vi "PWM.vi"(9 "Period (ms)":dbl=3.0, 10 "Duty Cycle":dbl format="%#_13g", 11 "Starting Tick Count":u32) -> (2 "Pwm value":bool, 3 "Starting Tick Count":u32)   [LabVIEW 2013]
doc: "Use this template to build a standard state machine design pattern. Each state executes code and determines which state to transition to. Contrast this design pattern with the User Interface Event Handler pattern, in which code executes in response to user actions. Contrast this design pattern also with the Queued Message Handler pattern, in which each message handling code can queue zero or more new messages."
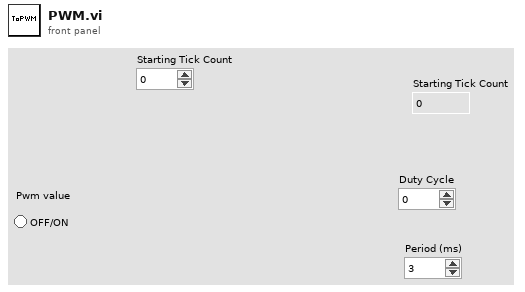
[diagram p1: front panel]
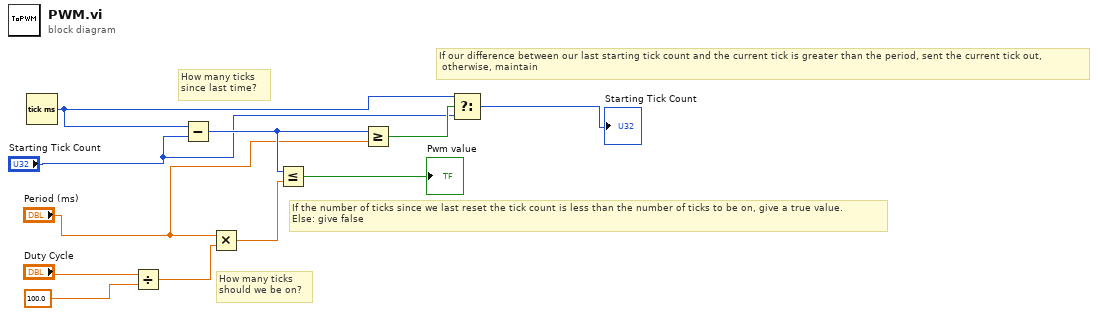
[diagram p0: block diagram]
diagram:
  # "If our difference between our last starting tick count and the current tick is greater than the period, sent the current tick out,\n otherwise, maintain"
  # "If the number of ticks since we last reset the tick count is less than the number of ticks to be on, give a true value.\nElse: give false"
  # "How many ticks \nsince last time?"
  # "How many ticks \nshould we be on?"
  n1 = Tick Count (ms)() -> (millisecond timer value=w3:u32)
  n2 = Divide(x="Duty Cycle", y=100.0) -> (x/y=w9:dbl)
  n3 = Subtract(x=w3, y="Starting Tick Count") -> (x-y=w6:u32)
  n4 = Multiply(x="Period (ms)", y=w9) -> (x*y=w8:dbl)
  n5 = Less Or Equal?(x=w6, y=w8) -> (x <= y?=→"Pwm value":bool)
  n6 = Greater Or Equal?(x=w6, y="Period (ms)") -> (x >= y?=w4:bool)
  n7 = Select(t=w3, s=w4, f="Starting Tick Count") -> (s? t:f=→"Starting Tick Count":u32)
